vi "DeleteReferences.vi"(8 "error in (no error)":errorcluster, 11 "data in":T1) -> (0 "error out":errorcluster)   [LabVIEW 2017, in "DataFlow.lvlib"]
uses:
  <vilib>/addons/InsightCM/Devices/Shared/Common/DataFlow/DataFlow.lvlib
  <vilib>/addons/InsightCM/Devices/Shared/Common/DataFlow/controls/Data.ctl
  <vilib>/addons/InsightCM/Utilities/DataAccessors/controls/wfmSGL_DVR.ctl
  <vilib>/addons/PointValueMap/controls/PointMap.ctl
  <vilib>/addons/InsightCM/Devices/Shared/Common/DataFlow/controls/Type.ctl
  <vilib>/addons/PointValueMap/subVIs/Point_Read_variant.vi
  <vilib>/addons/PointValueMap/PointValueMap.lvlib
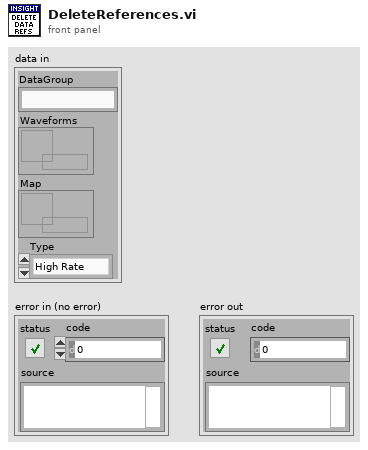
[diagram p1: front panel]
types:
  T1 = typedef "DataFlow.lvlib/Data.ctl" = cluster{"DataGroup":string, "Waveforms":T2, "Map":T3, "Type":T4}
  T2 = typedef "wfmSGL_DVR.ctl" = refnum<data-value>
  T3 = typedef "PointValueMap.lvlib/PointMap.ctl" = refnum<data-value>
  T4 = typedef "DataFlow.lvlib/Type.ctl" = enum16{"High Rate", "Low Rate", "Burst Mode"}
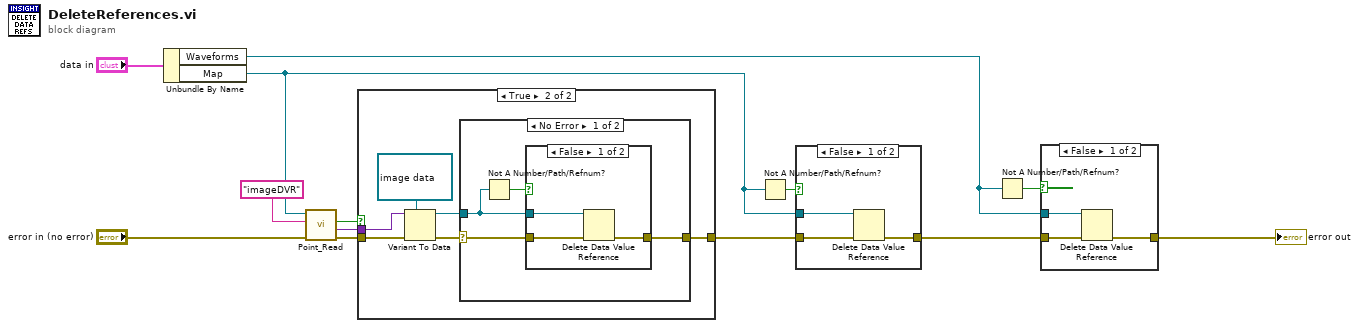
[diagram p0: block diagram]
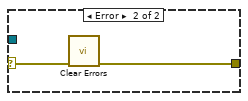
[diagram p4: hidden frame]
diagram:
  n1 = Unbundle By Name("data in") -> ("Waveforms"=w11:T2, "Map"=w6:T3)
  n2 = call-poly <vilib>:"Point_Read.vi"("Error In"="error in (no error)", "Tag"="imageDVR", "Map"=w6) -> ("Error Out"=w3:errorcluster, "Value"=w2:variant, "Found?"=w5:bool)  [unwired: 3 in, 3 out]
  n3 = case shown="True" w5 {
    tunnel: [w14 w17] -> w4
    tunnel: w3 -> [w14 w18]
    tunnel: w2 -> [_ w19]
    frame False {
    }
    frame True {
      n4 = Variant To Data(error in=w18, type=refnum<data-value> refnum ("data value reference"), Variant=w19) -> (data=w16:refnum<data-value>, error out=w15:errorcluster)
      n5 = case shown="No Error" w15 {
        selector: w15 -> [w21 w30]
        tunnel: [w24 w29] -> w17
        tunnel: w16 -> [w23 _]
        frame No Error {
          n6 = Not A Number/Path/Refnum?(number/path/refnum=w23) -> (NaN/Path/Refnum?=w22:bool)
          n7 = case shown="False" w22 {
            tunnel: w21 -> [w27 w28]
            tunnel: [w26 w28] -> w24
            tunnel: w23 -> [w25 _]
            frame False {
              n8 = Delete Data Value Reference(data value reference=w25, error in=w27) -> (error out=w26:errorcluster)  [unwired: 1 out]
            }
            frame True {
            }
          }
        }
        frame Error {
          n9 = call <vilib>:"Clear Errors.vi"("error in (no error)"=w30) -> ("error out"=w29:errorcluster)  [unwired: 5 in, 1 out]
        }
      }
    }
  }
  n10 = Not A Number/Path/Refnum?(number/path/refnum=w6) -> (NaN/Path/Refnum?=w13:bool)
  n11 = case shown="False" w13 {
    tunnel: w4 -> [w33 w34]
    tunnel: [w32 w34] -> w9
    tunnel: w6 -> [w31 _]
    frame False {
      n12 = Delete Data Value Reference(data value reference=w31, error in=w33) -> (error out=w32:errorcluster)  [unwired: 1 out]
    }
    frame True {
    }
  }
  n13 = Not A Number/Path/Refnum?(number/path/refnum=w11) -> (NaN/Path/Refnum?=w12:bool)
  n14 = case shown="False" w12 {
    tunnel: w9 -> [w37 w38]
    tunnel: [w36 w38] -> w10
    tunnel: w11 -> [w35 _]
    frame False {
      n15 = Delete Data Value Reference(data value reference=w35, error in=w37) -> (error out=w36:errorcluster)  [unwired: 1 out]
    }
    frame True {
    }
  }
  "error out" <- w10
